vi "test_parse generic data with strings.vi"() -> ()   [LabVIEW 2020]
uses:
  <vilib>/AdvancedString/1D String Array to Delimited String.vi
  Users/JKI/Desktop/parse generic data with strings.vi/ed5590e3-c1f7-48d3-8ff7-d9ee3b767263.vi
  Users/JKI/Desktop/parse generic data with strings.vi/a5b7f845-be68-4c9a-ad6c-83d99c3db13b.vi
  Users/JKI/Desktop/parse generic data with strings.vi/88aeaf81-e89a-43ae-9e76-8fa1d67f37f9.vi
  Users/JKI/Desktop/parse generic data with strings.vi/cfe8da2e-4b12-4f12-b932-2a0625bc18f4.vi
  Users/JKI/Desktop/parse generic data with strings.vi/4609e594-e62c-4725-984f-cc1e22b184a7.vi
  Users/JKI/Desktop/parse generic data with strings.vi/01dc9cd7-1da2-47da-a8d7-1150ed450fbb.vi
  Users/JKI/Desktop/parse generic data with strings.vi/1a77bec5-1a35-43cc-b640-5a18640e21d6.vi
  Users/JKI/Desktop/parse generic data with strings.vi/b5184ad7-a107-4c31-b670-5c4db2b6eaac.vi
  Users/JKI/Desktop/parse generic data with strings.vi/d7255a6e-ae9a-40df-94e1-f7199c397288.vi
  <vilib>/JDP Science/JSONtext/Make JSON Array.vi
  Users/JKI/Desktop/parse generic data with strings.vi/5171cadf-4f01-4683-b61d-c49ebc1a03d1.vi
  Users/JKI/Desktop/parse generic data with strings.vi/bd4dc24f-41f2-4310-95cd-0bf77e7af417.vi
  <vilib>/LabVIEW Open Source Project/Epoch Date & Time/epoch.UNIX/Epoch.UNIX.lvclass
  C:/Program Files/National Instruments/LabVIEW 2020/vi.lib/LabVIEW Open Source Project/Epoch Date & Time/epoch/Epoch.lvclass
  <userlib>/_OpenG.lib/lvdata/lvdata.llb/Get Data Name__ogtk.vi
  <userlib>/_OpenG.lib/lvdata/lvdata.llb/Cluster to Array of VData__ogtk.vi
  <vilib>/LabVIEW Open Source Project/Epoch Date & Time/Get Epoch Time.vi
  <vilib>/JDP Science/JSONtext/Variant to JSON Text.vi
  <vilib>/JDP Science/JSONtext/Set Item.vi
  <userlib>/_OpenG.lib/lvdata/lvdata.llb/Get TDEnum from Data__ogtk.vi
  <vilib>/Utility/error.llb/Error Cluster From Error Code.vi
  <vilib>/JDP Science/JSONtext/support/Format JSON Array Text.vi
  <vilib>/JDP Science/JSONtext/LVClass Serializer/JSONtext LVClass Serializer.lvclass
panel:
  out "error out":errorcluster
  out "Time Taken":dbl
  in  "Time Stamp (now: system time)":timestamp format="%<%x %.3X>T"
  in  "dataSourceRid":string="RID1234abce!\"£$"
  in  "Owning Cluster":T1={"1"=1, "Status"="", "Nested 1"={"2"=2, "3"=3, "Nested 2"={"4"=4, "5"=5, "1"=1.0, "qwe"=FALSE}, "qwe"=FALSE, "Status"="", "6"=6}}
  out "JSON":string
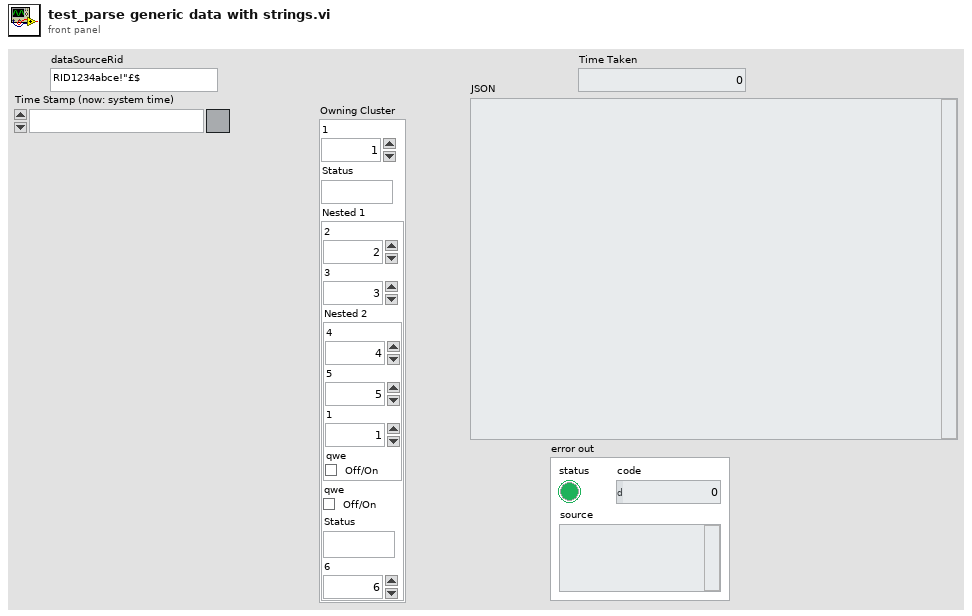
[diagram p1: front panel]
types:
  T1 = cluster{"1":i32, "Status":string, "Nested 1":cluster{"2":i32, "3":i8, "Nested 2":cluster{"4":i32, "5":i32, "1":dbl, "qwe":bool}, "qwe":bool, "Status":string, "6":i32}}
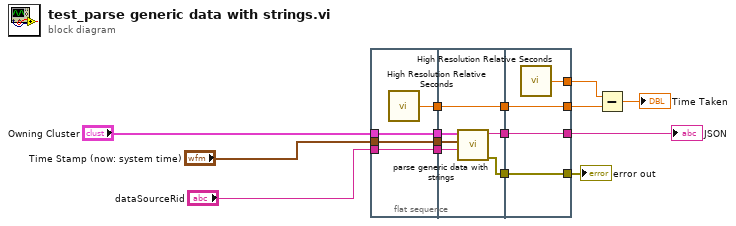
[diagram p0: block diagram]
diagram:
  n1 = flat-sequence {
    tunnel: "Time Stamp (now: system time)" -> [w17]
    tunnel: "Owning Cluster" -> [w18]
    tunnel: "dataSourceRid" -> [w19]
    tunnel: [w19] -> w11
    tunnel: [w18] -> w10
    tunnel: [w17] -> w9
    tunnel: [w16] -> w7
    tunnel: [w23] -> w12
    tunnel: w11 -> [w25]
    tunnel: w10 -> [w24]
    tunnel: w9 -> [w22]
    tunnel: [w21] -> w8
    tunnel: w7 -> [w21]
    tunnel: [w20] -> w2
    tunnel: [w29] -> w3
    tunnel: w12 -> [w29]
    tunnel: [w28] -> w6
    tunnel: w8 -> [w28]
    tunnel: [w27] -> w5
    tunnel: [w26] -> w1
    tunnel: w2 -> [w26]
    frame #0 {
      n2 = call <vilib>:"High Resolution Relative Seconds.vi"() -> ("relative seconds"=w16:dbl)
    }
    frame #1 {
      n3 = call "parse generic data with strings.vi"("dataSourceRid"=w25, "Time Stamp (now: system time)"=w22, "Data Cluster"=w24) -> ("error out"=w20:errorcluster, "JSON"=w23:string)  [unwired: 7 in]
    }
    frame #2 {
      n4 = call <vilib>:"High Resolution Relative Seconds.vi"() -> ("relative seconds"=w27:dbl)
    }
  }
  n5 = Subtract(x=w5, y=w6) -> (x-y=→"Time Taken":dbl)
  "JSON" <- w3
  "error out" <- w1
